vi "Read CAN FIFO.vi"(8 "error in (no error)":errorcluster, 9 "Timeout (ms)":i32, 11 "CIFTag in":refnum<class "CIF_NIChn_FifoCAN.lvclass">) -> (0 "error out":errorcluster, 1 "timed out?":bool, 2 "Data out":u8[](array[numeric]), 3 "CIFTag out":refnum<class "CIF_NIChn_FifoCAN.lvclass">, 4 "Header":T1)   [LabVIEW 2021, in "CIF_NIChn_FifoCAN.lvclass"]
uses:
  CIF_NIChn_FifoCAN.lvclass
  ChannelCommon/typedef/FIFO Header.ctl
  CIF_NIChn_FifoCAN.lvclass/CIF_NIChn_FifoCAN.ctl
  ChannelCommon/ChannelCommon.lvlib
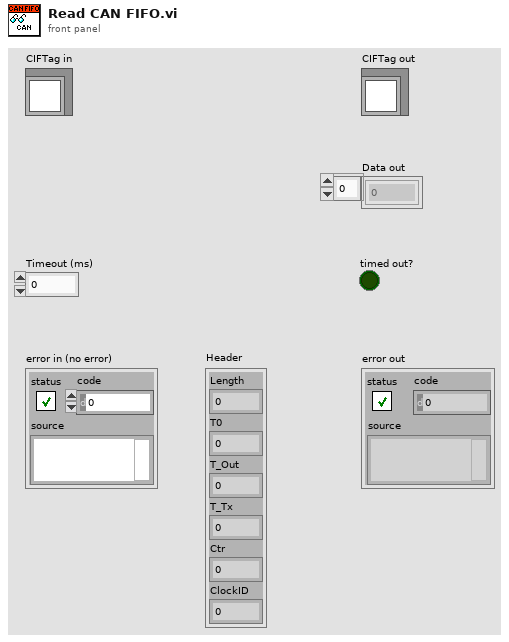
[diagram p1: front panel]
types:
  T1 = typedef "ChannelCommon.lvlib/FIFO Header.ctl" = cluster{"Length":u64, "T0":i64, "T_Out":i64, "T_Tx":i64, "Ctr":u64, "ClockID":u8}
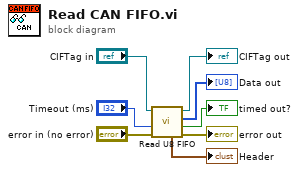
[diagram p0: block diagram]
diagram:
  n1 = call-dynamic "Read U8 FIFO.vi"("error in (no error)"="error in (no error)", "Timeout (ms)"="Timeout (ms)", "CIFFIFO in"="CIFTag in") -> ("error out"=→"error out":errorcluster, "timed out?"=→"timed out?":bool, "Data out"=→"Data out":u8[], "CIFFIFO out"=→"CIFTag out":refnum<class "CIF_NIChn_FifoCAN.lvclass">, "Header"=→"Header":T1)  [unwired: 4 in]
